vi "Execute.vi"(10 "Test Runner V2 in":refnum<class "Runnable.lvclass">, 11 "Single Thread Test Runner In":refnum<class "Single Thread Test Runner.lvclass">) -> ()   [LabVIEW 2020, in "Single Thread Test Runner.lvclass"]
uses:
  Single Thread Test Runner.lvclass
  Runnable.lvclass
  Core/Result/Result.ctl
  Core/Result/Status.ctl
  Core/Result/Type.ctl
  Single Thread Test Runner.lvclass/Single Thread Test Runner.ctl
  Result Observer/Result Observer.lvclass
  Core/Result/Result.lvlib
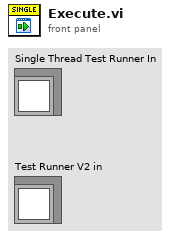
[diagram p1: front panel]
types:
  T1 = typedef "Result.lvlib/Result.ctl" = cluster{"Name":string, "Description":string, "Status":T2, "Result Type":T3, "Execution Time":dbl, "Data":cluster{"Expected":variant, "Actual":variant, "Delta":variant}}
  T2 = typedef "Result.lvlib/Status.ctl" = enum16{"", "Passed", "Failed", "Error", "Skipped", "Setup Error", "Broken", "Teardown Error"}
  T3 = typedef "Result.lvlib/Type.ctl" = enum16{"Test Case", "Test Suite", "Test Run", "Pass", "Fail", "Skip", "Pass if", "Fail if", "Pass if Error", "Fail if Error", "Pass if Equal", "Fail if Equal"}
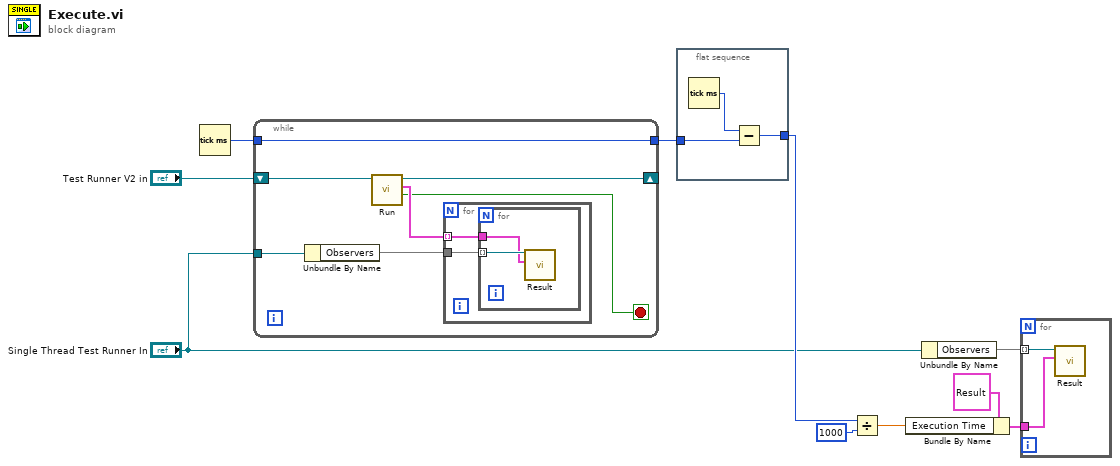
[diagram p0: block diagram]
diagram:
  n1 = Tick Count (ms)() -> (millisecond timer value=w7:u32)
  n2 = while {
    shift-right: [w15] -> _
    shift-left: "Test Runner V2 in" -> [w17]
    tunnel: "Single Thread Test Runner In" -> [w14]
    tunnel: [w11] -> w6
    tunnel: w7 -> [w11]
    stop <- w13 stop-if-true
    n3 = Unbundle By Name(w14) -> ("Observers"=w12:set{refnum<class "Result Observer.lvclass">})
    n4 = call-dynamic "Run.vi"("Runnable In"=w17) -> ("Done?"=w13:bool, "Results"=w16:T1[], "Runnable Out"=w15:refnum<class "Runnable.lvclass">)  [unwired: 7 in, 1 out]
    n5 = for {
      tunnel: w16 -> [w18] mode=indexing
      tunnel: w12 -> [w19]
      n6 = for {
        tunnel: w19 -> [w21] mode=indexing
        tunnel: w18 -> [w20]
        n7 = call-dynamic "Result.vi"("Result"=w20, "Result Observer In"=w21) -> ()  [unwired: 9 in, 1 out]
      }
    }
  }
  n8 = flat-sequence {
    tunnel: [w24] -> w9
    tunnel: w6 -> [w22]
    frame #0 {
      n9 = Tick Count (ms)() -> (millisecond timer value=w23:u32)
      n10 = Subtract(x=w23, y=w22) -> (x-y=w24:u32)
    }
  }
  n11 = Divide(x=w9, y=u32 1000) -> (x/y=w5:dbl)
  n12 = Bundle By Name(cluster=T1 {"Name"="", "Description"="", "Status"=enum."Passed", "Result Type"=enum."Test Run", "Execution Time"=0.0, "Data"={"Expected"=variant, "Actual"=variant, "Delta"=variant}} ("Result"), "Execution Time"=w5) -> (w2:T1)
  n13 = Unbundle By Name("Single Thread Test Runner In") -> ("Observers"=w4:set{refnum<class "Result Observer.lvclass">})
  n14 = for {
    tunnel: w4 -> [w26] mode=indexing
    tunnel: w2 -> [w25]
    n15 = call-dynamic "Result.vi"("Result"=w25, "Result Observer In"=w26) -> ()  [unwired: 9 in, 1 out]
  }
